vi "SetupLockIn.vi"(4 "Sensitivity (26: 1 V/uA)":i8(ring)=26 items=["Auto Gain"=-1, "2 nV/fA"=0, "5 nV/fA"=1, "10 nV/fA"=2, "20 nV/fA"=3, "50 nV/fA"=4, "100 nV/fA"=5, "200 nV/fA"=6, "500 nV/fA"=7, "1 uV/pA"=8, "2 uV/pA"=9, "5 uV/pA"=10, "10 uV/pA"=11, "20 uV/pA"=12, "50 uV/pA"=13, "100 uV/pA"=14, "200 uV/pA"=15, "500 uV/pA"=16, "1 mV/nA"=17, "2 mV/nA"=18, "5 mV/nA"=19, "10 mV/nA"=20, "20 mV/nA"=21, "50 mV/nA"=22, "100 mV/nA"=23, "200 mV/nA"=24, "500 mV/mA"=25, "1 V/uA"=26], 5 "Dynamic Reserve (2: Low Noise)":i8(ring)=2 items=["High Reserve"=0, "Normal"=1, "Low Noise"=2, "Auto Reserve"=-1], 6 "Sine Output Amplitude (1 V)":dbl=1.0, 7 "Reference Source (1: Internal)":u16(ring)=1 items=["External", "Internal"], 8 "Internal Reference Frequency (1000 Hz)":dbl=1000.0, 9 "Input Coupling (0: AC)":u16(ring) items=["AC", "DC"], 10 "Input Connection (0: Single-Ended Voltage)":u16(ring) items=["Single-Ended Voltage", "Differential Voltage", "1 MOhm Current Gain", "100 MOhm Current Gain"], 11 "VISA Refnum in":refnum<visa-resource-name>) -> (0 "error out":errorcluster, 2 "V_AC Amplitude (A)":dbl=1.0, 3 "VISA Refnum out":refnum<visa-resource-name>)   [LabVIEW 2012]
uses:
  Program Files/National Instruments/LabVIEW 2014/instr.lib/Stanford Research 830/Stanford Research 830.lvlib
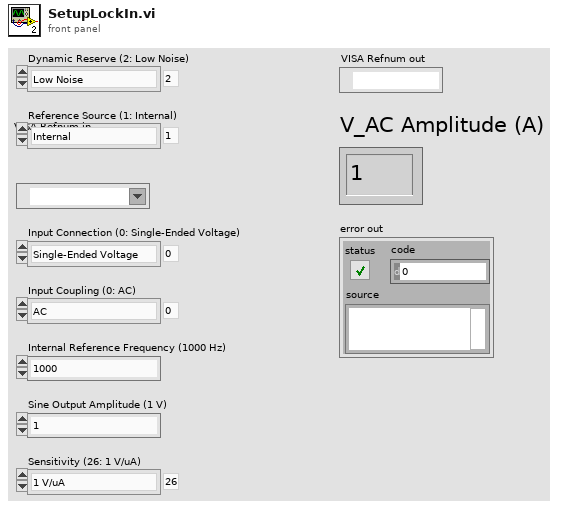
[diagram p1: front panel]
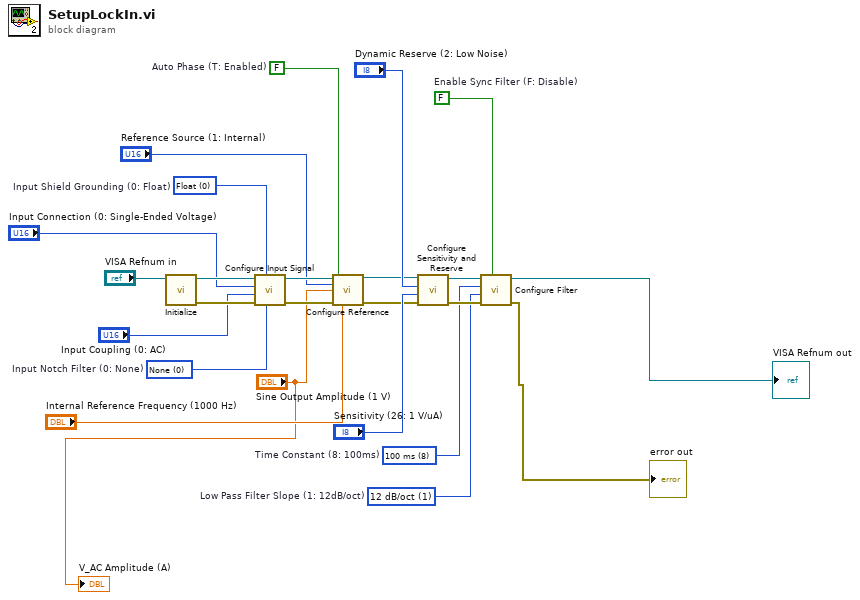
[diagram p0: block diagram]
diagram:
  w2 = u16 1 items=["6 dB/oct", "12 dB/oct", "18 db/oct", "24 dB/oct"]  # Low Pass Filter Slope (1: 12dB/oct)
  w3 = u16 8 items=["10 us", "30 us", "100 us", "300 us", "1 ms", "3 ms", "10 ms", "30 ms", "100 ms", "300 ms", "1 s", "3 s", "10 s", "30 s", "100 s", "300 s", "1 ks", "3 ks", "10 ks", "30 ks"]  # Time Constant (8: 100ms)
  w4 = FALSE  # Enable Sync Filter (F: Disable)
  w13 = FALSE  # Auto Phase (T: Enabled)
  w14 = u16 0 items=["None", "Line Notch", "2x Line Notch", "Both Notch Filters"]  # Input Notch Filter (0: None)
  w15 = u16 0 items=["Float", "Ground"]  # Input Shield Grounding (0: Float)
  n1 = call "Initialize.vi"("VISA resource name"="VISA Refnum in") -> ("error out"=w21:errorcluster, "VISA resource name out"=w20:refnum<visa-resource-name>)  [unwired: 9 in]
  n2 = call "Configure Input Signal.vi"("Input Notch Filter (0: None)"=w14, "Input Shield Grounding (0: Float)"=w15, "error in (no error)"=w21, "Input Coupling (0: AC)"="Input Coupling (0: AC)", "Input Connection (0: Single-Ended Voltage)"="Input Connection (0: Single-Ended Voltage)", "VISA resource name"=w20) -> ("error out"=w18:errorcluster, "VISA resource name out"=w19:refnum<visa-resource-name>)  [unwired: 4 in]
  n3 = call "Configure Reference.vi"("VISA resource name"=w19, "Auto Phase (T: Enabled)"=w13, "Reference Source (1: Internal)"="Reference Source (1: Internal)", "Sine Output Amplitude (1 V)"="Sine Output Amplitude (1 V)", "error in (no error)"=w18, "Internal Reference Frequency (1000 Hz)"="Internal Reference Frequency (1000 Hz)") -> ("VISA resource name out"=w10:refnum<visa-resource-name>, "error out"=w9:errorcluster)  [unwired: 8 in]
  n4 = call "Configure Sensitivity and Reserve.vi"("error in (no error)"=w9, "Sensitivity (-1: Auto gain)"="Sensitivity (26: 1 V/uA)", "Dynamic Reserve (-1: Auto Reserve)"="Dynamic Reserve (2: Low Noise)", "VISA resource name"=w10) -> ("error out"=w6:errorcluster, "VISA resource name out"=w5:refnum<visa-resource-name>)  [unwired: 6 in]
  n5 = call "Configure Filter.vi"("Enable Sync Filter (F: Disable)"=w4, "error in (no error)"=w6, "Low Pass Filter Slope (1: 12dB/oct)"=w2, "Time Constant (8: 100ms)"=w3, "VISA resource name"=w5) -> ("error out"=→"error out":errorcluster, "VISA resource name out"=→"VISA Refnum out":refnum<visa-resource-name>)  [unwired: 5 in]
  "V_AC Amplitude (A)" <- "Sine Output Amplitude (1 V)"
